vi "GetType.vi"(8 "error in (no error)":errorcluster, 11 "Configure Sample Clock [SC] Msg":refnum<class "Configure Sample Clock [SC] Msg.lvclass">) -> (0 "error out":errorcluster, 2 "Data Sample":variant, 3 "Configure Sample Clock [SC] Msg":refnum<class "Configure Sample Clock [SC] Msg.lvclass">)   [LabVIEW 2015, in "CS++Fgen.lvlib" / "Configure Sample Clock [SC] Msg.lvclass"]
doc: "This VI delivers a sample of the data type format the message expects."
uses:
  Configure Sample Clock [SC] Msg.lvclass
  Configure Sample Clock [SC] Msg.lvclass/Configure Sample Clock [SC] Msg.ctl
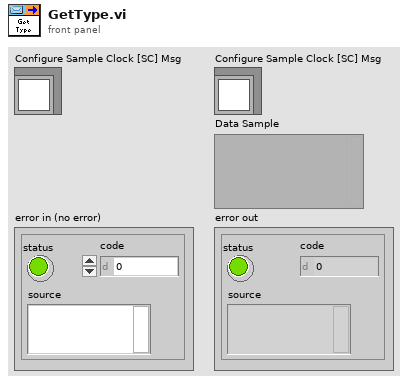
[diagram p1: front panel]
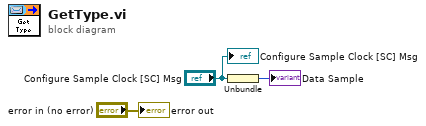
[diagram p0: block diagram]
diagram:
  n1 = Unbundle("Configure Sample Clock [SC] Msg") -> (→"Data Sample":i32)
  "error out" <- "error in (no error)"
  "Configure Sample Clock [SC] Msg" <- "Configure Sample Clock [SC] Msg"
